vi "G#Object_GenericOpen.vi"(0 "reference in":refnum<class "G#Object.lvclass">, 4 "timeout in ms (-1)":i32=-1, 5 "error in (no error)":errorcluster) -> (14 "reference out":refnum<class "G#Object.lvclass">, 15 "external creator running?":bool, 19 "error out":errorcluster)   [LabVIEW 2020, in "G#Object.lvclass"]
doc: "Runs the \"G#Object_Open.vi\" of the class. Override this method if the external create process is running, an event will be sent to let this process create and own the VI (and everything this might create). This way LabVIEW garbage collector will not clear the resources until it is destroyed or the garbage collector runs."
uses:
  G#Object.lvclass
  utils/G#Object_EventType.ctl
  utils/G#Object_ObjectInfoType.ctl
  utils/G#Object_CreateMethod.ctl
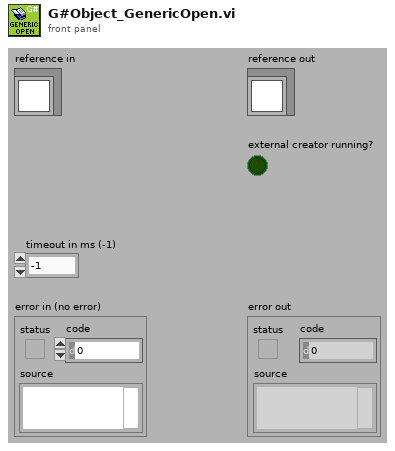
[diagram p1: front panel]
types:
  T1 = typedef "G#Object.lvclass/G#Object_ObjectInfoType.ctl" = cluster{"ObjectName":string, "ObjectID":u32, "Users":i32, "Counter":bool, "AttributeRefs":u32[], "FullClassName":string, "ClassName":string, "CreateMethod":T2, "GenericDestructorExists":bool, "Owner":string}
  T2 = typedef "G#Object.lvclass/G#Object_CreateMethod.ctl" = enum16{"Create", "Create or look up existing", "Look up existing"}
  T3 = typedef "G#Object.lvclass/G#Object_EventType.ctl" = enum16{"Created new", "Looked up existing", "Deleted", "Forced delete", "Not deleted", "Garbage collected", "Cleared", "User", "Error", "External create object", "External create class attributes", "Created class attributes", "Run constructor", "Run constructor done", "Run open method", "Run open method done"}
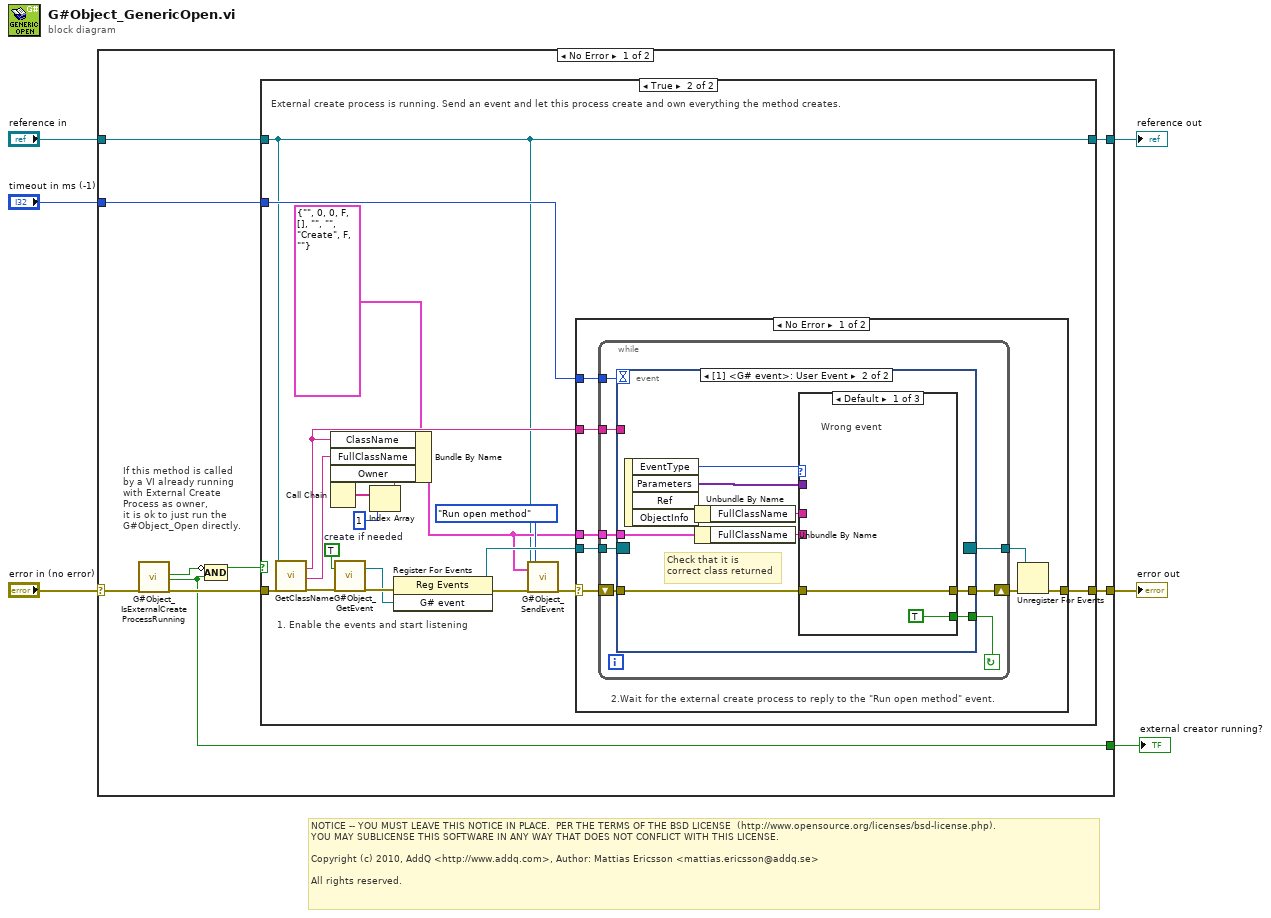
[diagram p0: block diagram]
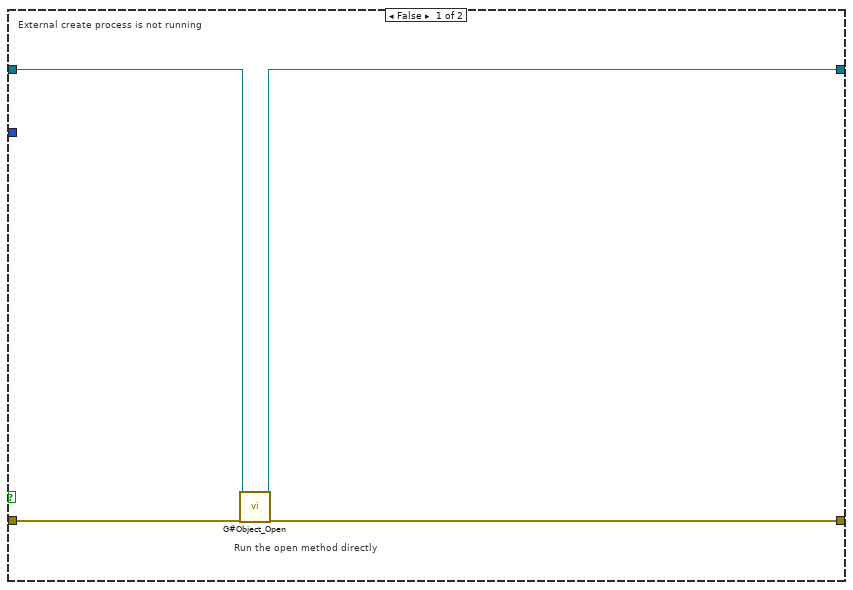
[diagram p2: hidden frame]
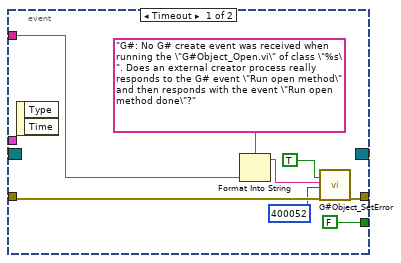
[diagram p3: hidden frame]
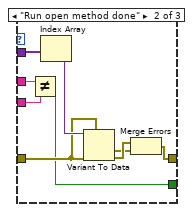
[diagram p4: hidden frame]
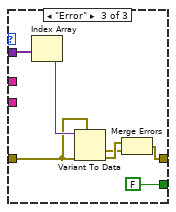
[diagram p5: hidden frame]
diagram:
  # "NOTICE -- YOU MUST LEAVE THIS NOTICE IN PLACE.  PER THE TERMS OF THE BSD LICENSE  (http://www.opensource.org/licenses/bsd-license.php).\nYOU MAY SUBLICENSE THIS SOFTWARE IN ANY WAY THAT DOES NOT CONFLICT WITH THIS LICENSE.\n\nCopyright (c) 2010, AddQ <http://www.addq.com>, Author: Mattias Ericsson <mattias.ericsson@addq.se>\n\nAll rights reserved."
  n1 = case shown="No Error" "error in (no error)" {
    selector: "error in (no error)" -> [w11 w92]
    tunnel: [w12 w92] -> w5
    tunnel: [w15 w91] -> w4
    tunnel: "timeout in ms (-1)" -> [w14 _]
    tunnel: "reference in" -> [w13 w91]
    tunnel: [w8 _] -> w1
    frame No Error {
      # "If this method is called\nby a VI already running\nwith External Create\nProcess as owner,\nit is ok to just run the\nG#Object_Open directly."
      n2 = call "G#Object_IsExternalCreateProcessRunning.vi"("error in (no error)"=w11) -> ("owned by external process?"=w10:bool, "external create process running?"=w8:bool, "error out"=w9:errorcluster)  [unwired: 15 in, 1 out]
      n3 = Compound Arithmetic op=AND(invert w10, w8) -> (w7:bool)
      n4 = case shown="True" w7 {
        tunnel: [w17 w25] -> w15
        tunnel: w13 -> [w18 w25]
        tunnel: w14 -> [_ w31]
        tunnel: w9 -> [w19 w28]
        tunnel: [w16 w24] -> w12
        frame False {
          # "External create process is not running"
          # "Run the open method directly"
          n5 = call-dynamic "G#Object_Open.vi"("reference in"=w18, "error in (no error)"=w19) -> ("reference out"=w17:refnum<class "G#Object.lvclass">, "error out"=w16:errorcluster)  [unwired: 16 in]
        }
        frame True {
          w36 = TRUE  # create if needed
          # "External create process is running. Send an event and let this process create and own everything the method creates."
          # "1. Enable the events and start listening"
          n6 = call-dynamic "GetClassName.vi"("reference in"=w25, "error in (no error)"=w28) -> ("class name"=w30:string, "full class name"=w32:string, "error out"=w29:errorcluster)  [unwired: 13 in, 2 out]
          n7 = Call Chain() -> (call chain=w23:string[])
          n8 = call "G#Object_GetEvent.vi"("create if needed (T)"=w36, "error in (no error)"=w29) -> ("G# event"=w35:refnum<user-event>, "error out"=w38:errorcluster)  [unwired: 13 in, 3 out]
          n9 = Index Array(array=w23, index=1) -> (element=w21:string)
          n10 = Bundle By Name(cluster=T1 {"ObjectName"="", "ObjectID"=0, "Users"=0, "Counter"=FALSE, "AttributeRefs"=[], "FullClassName"="", "ClassName"="", "CreateMethod"=enum."Create", "GenericDestructorExists"=FALSE, "Owner"=""} ("ObjectInfo"), "ClassName"=w30, "FullClassName"=w32, "Owner"=w21) -> (w27:T1)
          n11 = register-events(error in=w38, w35) -> (reference out=w37:refnum<event-registration>, error out=w34:errorcluster)  [unwired: 1 in]
          n12 = call "G#Object_SendEvent.vi"("reference in"=w25, "object info extended"=w27, "error in (no error)"=w34, "G# event type"=G#Object_EventType."Run open method") -> ("error out"=w20:errorcluster)  [unwired: 15 in]
          n13 = case shown="No Error" w20 {
            selector: w20 -> [w39 w90]
            tunnel: w37 -> [w46 _]
            tunnel: w31 -> [w43 _]
            tunnel: w30 -> [w42 _]
            tunnel: w27 -> [w41 _]
            tunnel: [w40 w90] -> w24
            frame No Error {
              # "2.Wait for the external create process to reply to the \"Run open method\" event."
              n14 = while {
                tunnel: w46 -> [w54]
                shift-right: [w52] -> w45
                shift-left: w39 -> [w53]
                tunnel: [w50] -> w44
                tunnel: w43 -> [w49]
                tunnel: w42 -> [w48]
                tunnel: w41 -> [w47]
                stop <- w51 continue-if-true
                n15 = event shown="[1] <G# event>: User Event" {
                  selector: w54 -> [_ _]
                  dyn-events: [_ _] -> w50
                  timeout: w49 -> [_ _]
                  tunnel: w53 -> [w60 w70]
                  tunnel: [w61 w68] -> w52
                  tunnel: [FALSE w67] -> w51
                  tunnel: w48 -> [w56 _]
                  tunnel: w47 -> [_ w64]
                  event Timeout {
                    n16 = event-data() -> ()  [unwired: 1 in, 2 out]
                    n17 = Format Into String(format string="G#: No G# create event was received when running the \"G#Object_Open.vi\" of class \"%s\". Does an external creator process really responds to the G# event \"Run open method\" and then responds with the event \"Run open method done\"?" ("source"), w56) -> (resulting string=w57:string)  [unwired: 2 in, 1 out]
                    n18 = call "G#Object_SetError.vi"("error (F)"=TRUE ("error"), "source"=w57, "code"=400052, "error in (no error)"=w60) -> ("error out"=w61:errorcluster)  [unwired: 15 in]
                  }
                  event User Event {
                    # "Check that it is\ncorrect class returned"
                    n19 = event-data() -> ("EventType"=w71:T3, "Parameters"=w69:variant[], "ObjectInfo"=w66:T1)  [unwired: 1 in, 1 out]
                    n20 = Unbundle By Name(w66) -> ("FullClassName"=w63:string)
                    n21 = Unbundle By Name(w64) -> ("FullClassName"=w65:string)
                    n22 = case shown="Default" w71 {
                      tunnel: w70 -> [w73 w80 w87]
                      tunnel: w69 -> [_ w82 w89]
                      tunnel: [w73 w76 w86] -> w68
                      tunnel: [TRUE w77 FALSE] -> w67
                      tunnel: w63 -> [_ w79 _]
                      tunnel: w65 -> [_ w78 _]
                      frame Default {
                        # "Wrong event"
                      }
                      frame "Run open method done" {
                        n23 = Not Equal?(x=w79, y=w78) -> (x != y?=w77:bool)
                        n24 = Index Array(array=w82) -> (element=w81:variant)  [unwired: 1 in]
                        n25 = Variant To Data(error in=w80, type=w80, Variant=w81) -> (data=w74:errorcluster, error out=w75:errorcluster)
                        n26 = Merge Errors(w75, w74) -> (w76:errorcluster)
                      }
                      frame "Error" {
                        n27 = Index Array(array=w89) -> (element=w88:variant)  [unwired: 1 in]
                        n28 = Variant To Data(error in=w87, type=w87, Variant=w88) -> (data=w83:errorcluster, error out=w84:errorcluster)
                        n29 = Merge Errors(w84, w83) -> (w86:errorcluster)
                      }
                    }
                  }
                }
              }
              n30 = Unregister For Events(event registration refnum=w44, error in=w45) -> (error out=w40:errorcluster)
            }
            frame Error {
            }
          }
        }
      }
    }
    frame Error {
    }
  }
  "error out" <- w5
  "reference out" <- w4
  "external creator running?" <- w1
